vi "TraverseGObj.vi"(1 "Input":cluster{"Name":string, "Ctrl":refnum<vi>}[](array[cluster]), 2 "Prefix":string, 3 "GObj Reference":refnum<vi>) -> (0 "Output":cluster{"Name":string, "Ctrl":refnum<vi>}[](array[cluster]))   [LabVIEW 2014]
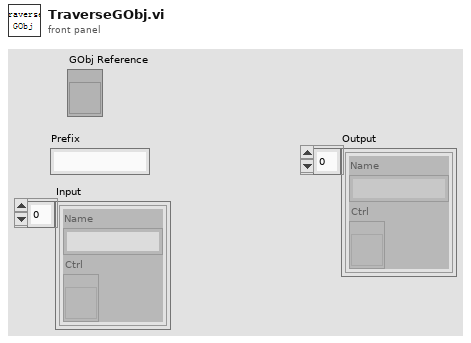
[diagram p1: front panel]
types:
  T1 = cluster{"Name":string, "GObj Reference":refnum<vi>}[]
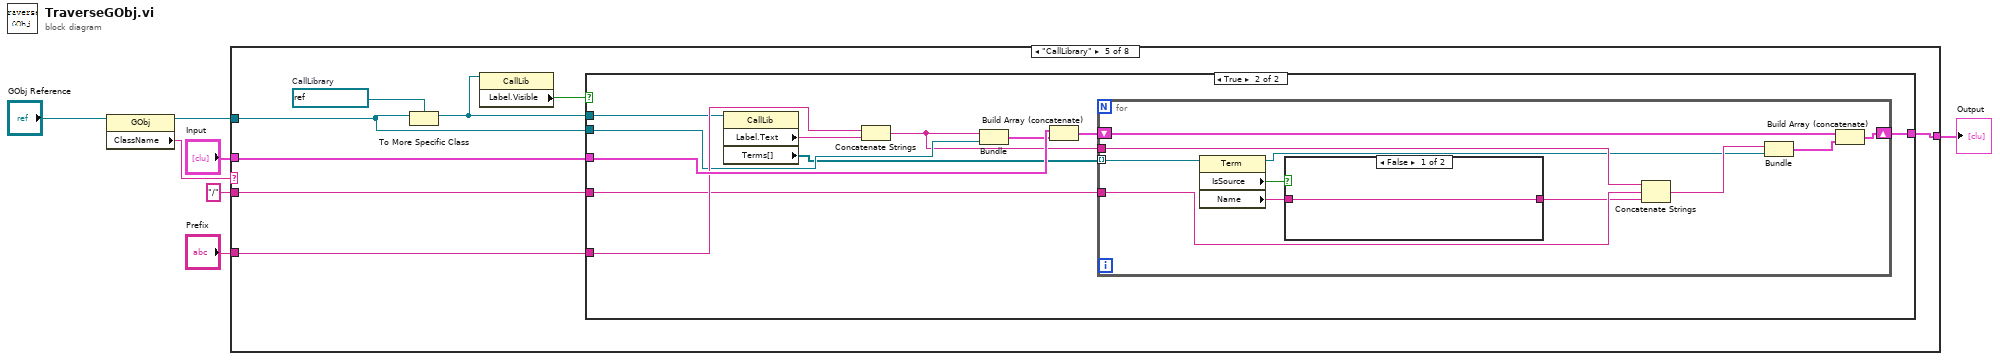
[diagram p0: block diagram]
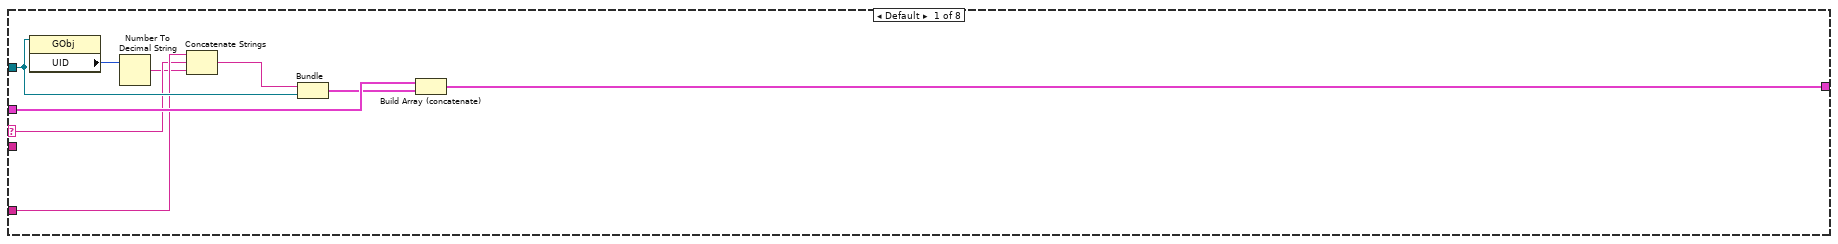
[diagram p2: hidden frame]
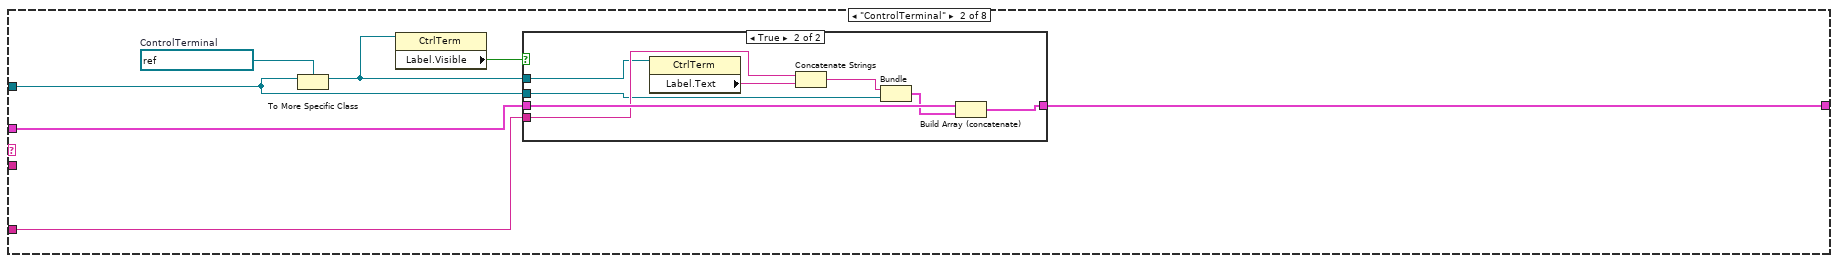
[diagram p3: hidden frame]
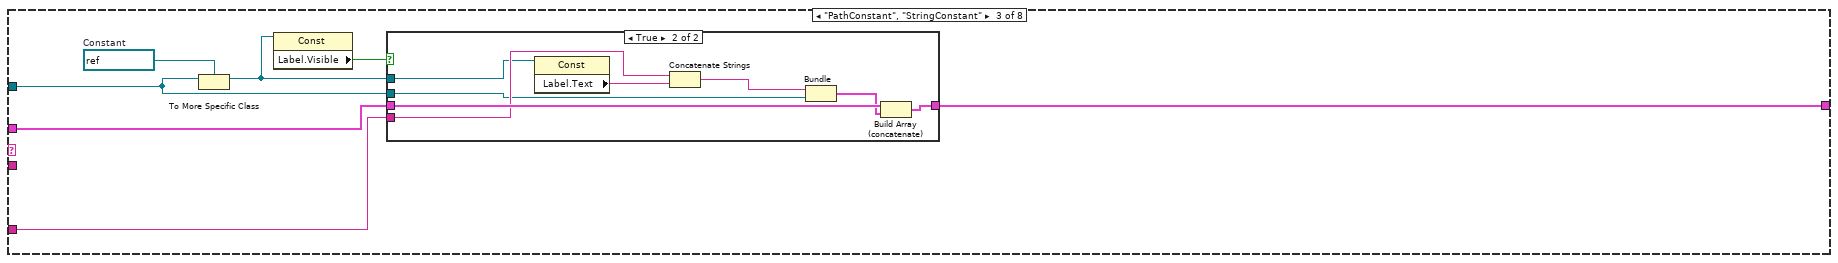
[diagram p5: hidden frame]
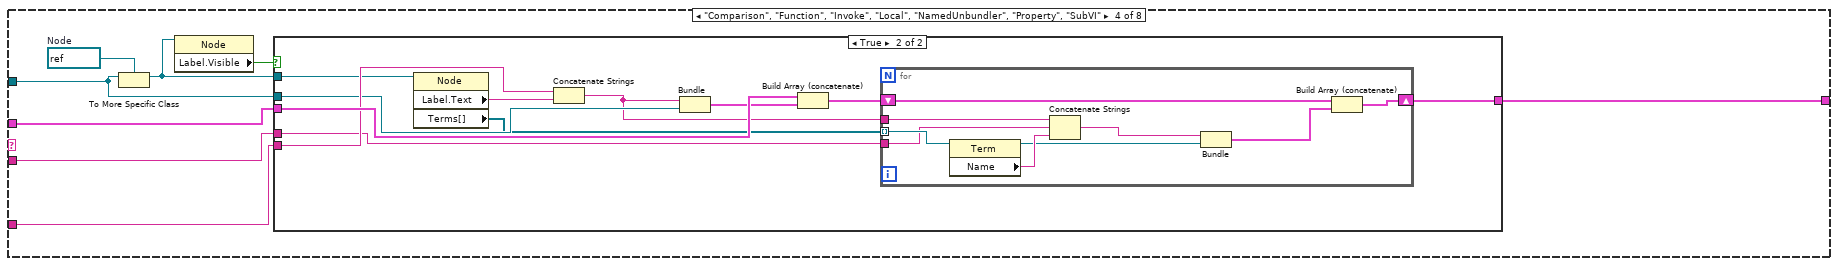
[diagram p7: hidden frame]
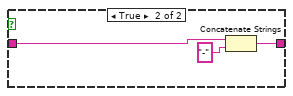
[diagram p10: hidden frame]
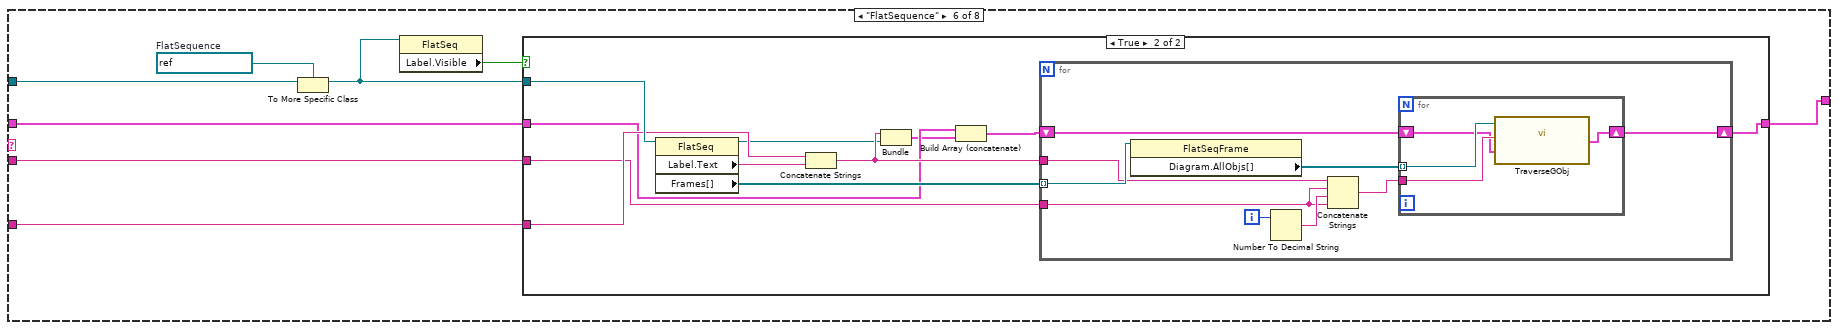
[diagram p11: hidden frame]
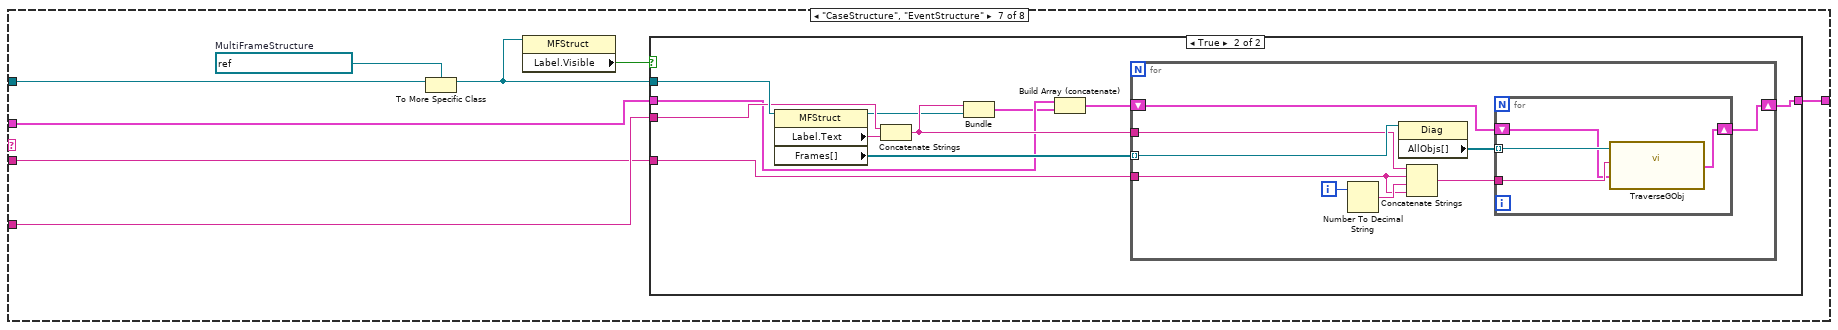
[diagram p13: hidden frame]
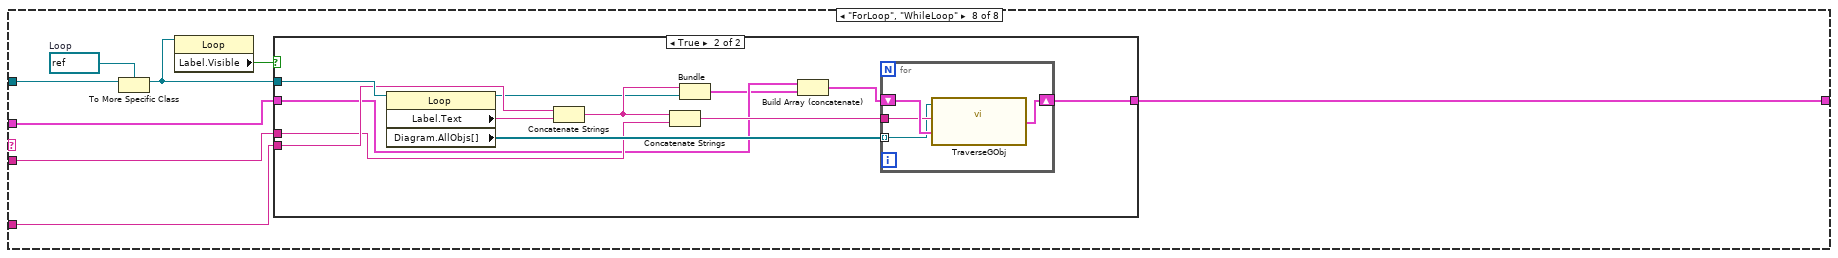
[diagram p15: hidden frame]
diagram:
  n1 = property on="Property Node" class="GObj"(reference="GObj Reference") -> (reference out=w6:refnum<vi>, "ClassName"=w7:string)  [unwired: 1 in, 1 out]
  n2 = case shown="\"CallLibrary\"" w7 {
    selector: w7 -> [w9 _ _ _ _ _ _ _]
    tunnel: w6 -> [w14 w19 w35 w52 w81 w120 w153 w186]
    tunnel: "Input" -> [w16 w23 w39 w56 w85 w118 w151 w185]
    tunnel: "Prefix" -> [w11 w21 w37 w54 w83 w117 w150 w184]
    tunnel: [w12 w22 w38 w55 w84 w116 w149 w183] -> w3
    tunnel: "/" ("string") -> [_ _ _ w49 w78 w115 w148 w181]
    frame Default {
      n3 = property class="GObj"(reference=w14) -> ("UID"=w13:i32)  [unwired: 1 in, 2 out]
      n4 = Number To Decimal String(number=w13) -> (decimal integer string=w8:string)  [unwired: 1 in]
      n5 = Concatenate Strings(w11, w9, w8) -> (w10:string)
      n6 = Bundle(w10, "GObj Reference"=w14) -> (w15:cluster{string, "GObj Reference":refnum<vi>})  [unwired: 1 in]
      n7 = Build Array (concatenate)(w16, w15) -> (w12:T1)
    }
    frame "ControlTerminal" {
      w20 = refnum<vi> refnum  # ControlTerminal
      n8 = To More Specific Class(target class=w20, reference=w19) -> (specific class reference=w18:refnum<vi>)  [unwired: 1 in, 1 out]
      n9 = property class="CtrlTerm"(reference=w18) -> ("Label.Visible"=w17:bool)  [unwired: 1 in, 2 out]
      n10 = case shown="True" w17 {
        tunnel: w23 -> [w24 w32]
        tunnel: [w24 w30] -> w22
        tunnel: w21 -> [_ w29]
        tunnel: w18 -> [_ w27]
        tunnel: w19 -> [_ w25]
        frame False {
        }
        frame True {
          n11 = property class="CtrlTerm"(reference=w27) -> ("Label.Text"=w26:string)  [unwired: 1 in, 2 out]
          n12 = Concatenate Strings(w29, w26) -> (w28:string)
          n13 = Bundle(w28, "GObj Reference"=w25) -> (w31:cluster{string, "GObj Reference":refnum<vi>})  [unwired: 1 in]
          n14 = Build Array (concatenate)(w32, w31) -> (w30:T1)
        }
      }
    }
    frame "PathConstant", "StringConstant" {
      w36 = refnum<vi> refnum  # Constant
      n15 = To More Specific Class(target class=w36, reference=w35) -> (specific class reference=w33:refnum<vi>)  [unwired: 1 in, 1 out]
      n16 = property class="Const"(reference=w33) -> ("Label.Visible"=w34:bool)  [unwired: 1 in, 2 out]
      n17 = case shown="True" w34 {
        tunnel: w39 -> [w40 w48]
        tunnel: [w40 w46] -> w38
        tunnel: w37 -> [_ w45]
        tunnel: w33 -> [_ w43]
        tunnel: w35 -> [_ w41]
        frame False {
        }
        frame True {
          n18 = property class="Const"(reference=w43) -> ("Label.Text"=w42:string)  [unwired: 1 in, 2 out]
          n19 = Concatenate Strings(w45, w42) -> (w44:string)
          n20 = Bundle(w44, "GObj Reference"=w41) -> (w47:cluster{string, "GObj Reference":refnum<vi>})  [unwired: 1 in]
          n21 = Build Array (concatenate)(w48, w47) -> (w46:T1)
        }
      }
    }
    frame "Comparison", "Function", "Invoke", "Local", "NamedUnbundler", "Property", "SubVI" {
      w53 = refnum<vi> refnum  # Node
      n22 = To More Specific Class(target class=w53, reference=w52) -> (specific class reference=w51:refnum<vi>)  [unwired: 1 in, 1 out]
      n23 = property class="Node"(reference=w51) -> ("Label.Visible"=w50:bool)  [unwired: 1 in, 2 out]
      n24 = case shown="True" w50 {
        tunnel: w56 -> [w57 w68]
        tunnel: [w57 w61] -> w55
        tunnel: w54 -> [_ w66]
        tunnel: w51 -> [_ w65]
        tunnel: w52 -> [_ w63]
        tunnel: w49 -> [_ w58]
        frame False {
        }
        frame True {
          n25 = property class="Node"(reference=w65) -> ("Label.Text"=w64:string, "Terms[]"=w60:refnum<vi>[])  [unwired: 1 in, 2 out]
          n26 = Concatenate Strings(w66, w64) -> (w59:string)
          n27 = Bundle(w59, "GObj Reference"=w63) -> (w67:cluster{string, "GObj Reference":refnum<vi>})  [unwired: 1 in]
          n28 = Build Array (concatenate)(w68, w67) -> (w62:T1)
          n29 = for {
            shift-right: [w69] -> w61
            shift-left: w62 -> [w71]
            tunnel: w60 -> [w77] mode=indexing
            tunnel: w59 -> [w76]
            tunnel: w58 -> [w75]
            n30 = property class="Term"(reference=w77) -> (reference out=w72:refnum<vi>, "Name"=w74:string)  [unwired: 1 in, 1 out]
            n31 = Concatenate Strings(w76, w75, w74) -> (w73:string)
            n32 = Bundle(w73, w72) -> (w70:cluster{string, refnum<vi>})  [unwired: 1 in]
            n33 = Build Array (concatenate)(w71, w70) -> (w69:T1)
          }
        }
      }
    }
    frame "CallLibrary" {
      w82 = refnum<vi> refnum  # CallLibrary
      n34 = To More Specific Class(target class=w82, reference=w81) -> (specific class reference=w80:refnum<vi>)  [unwired: 1 in, 1 out]
      n35 = property class="CallLib"(reference=w80) -> ("Label.Visible"=w79:bool)  [unwired: 1 in, 2 out]
      n36 = case shown="True" w79 {
        tunnel: w85 -> [w86 w97]
        tunnel: [w86 w90] -> w84
        tunnel: w83 -> [_ w95]
        tunnel: w80 -> [_ w94]
        tunnel: w81 -> [_ w92]
        tunnel: w78 -> [_ w87]
        frame False {
        }
        frame True {
          n37 = property class="CallLib"(reference=w94) -> ("Label.Text"=w93:string, "Terms[]"=w89:refnum<vi>[])  [unwired: 1 in, 2 out]
          n38 = Concatenate Strings(w95, w93) -> (w88:string)
          n39 = Bundle(w88, "GObj Reference"=w92) -> (w96:cluster{string, "GObj Reference":refnum<vi>})  [unwired: 1 in]
          n40 = Build Array (concatenate)(w97, w96) -> (w91:T1)
          n41 = for {
            shift-right: [w101] -> w90
            shift-left: w91 -> [w103]
            tunnel: w89 -> [w108] mode=indexing
            tunnel: w88 -> [w107]
            tunnel: w87 -> [w106]
            n42 = property class="Term"(reference=w108) -> (reference out=w104:refnum<vi>, "IsSource"=w100:bool, "Name"=w99:string)  [unwired: 1 in, 1 out]
            n43 = case shown="False" w100 {
              tunnel: w99 -> [w109 w112]
              tunnel: [w109 w110] -> w98
              frame False {
              }
              frame True {
                n44 = Concatenate Strings(w112, "-" ("string")) -> (w110:string)
              }
            }
            n45 = Concatenate Strings(w107, w106, w98) -> (w105:string)
            n46 = Bundle(w105, w104) -> (w102:cluster{string, refnum<vi>})  [unwired: 1 in]
            n47 = Build Array (concatenate)(w103, w102) -> (w101:T1)
          }
        }
      }
    }
    frame "FlatSequence" {
      w119 = refnum<vi> refnum  # FlatSequence
      n48 = To More Specific Class(target class=w119, reference=w120) -> (specific class reference=w114:refnum<vi>)  [unwired: 1 in, 1 out]
      n49 = property class="FlatSeq"(reference=w114) -> ("Label.Visible"=w113:bool)  [unwired: 1 in, 2 out]
      n50 = case shown="True" w113 {
        tunnel: w114 -> [_ w132]
        tunnel: w118 -> [w121 w124]
        tunnel: w117 -> [_ w131]
        tunnel: [w121 w128] -> w116
        tunnel: w115 -> [_ w127]
        frame False {
        }
        frame True {
          n51 = property class="FlatSeq"(reference=w132) -> (reference out=w125:refnum<vi>, "Label.Text"=w130:string, "Frames[]"=w129:refnum<vi>[])  [unwired: 1 in, 1 out]
          n52 = Concatenate Strings(w131, w130) -> (w126:string)
          n53 = Bundle(w126, w125) -> (w123:cluster{string, refnum<vi>})  [unwired: 1 in]
          n54 = Build Array (concatenate)(w124, w123) -> (w122:cluster{"Name":string, "Ctrl":refnum<vi>}[])
          n55 = for {
            tunnel: w129 -> [w141] mode=indexing
            tunnel: w126 -> [w140]
            shift-right: [w137] -> w128
            shift-left: w122 -> [w138]
            tunnel: w127 -> [w133]
            i -> [w135]
            n56 = property class="FlatSeqFrame"(reference=w141) -> ("Diagram.AllObjs[]"=w136:refnum<vi>[])  [unwired: 1 in, 2 out]
            n57 = Number To Decimal String(number=w135) -> (decimal integer string=w134:string)  [unwired: 1 in]
            n58 = Concatenate Strings(w140, w133, w134, w133) -> (w139:string)
            n59 = for {
              tunnel: w136 -> [w145] mode=indexing
              tunnel: w139 -> [w144]
              shift-right: [w142] -> w137
              shift-left: w138 -> [w143]
              n60 = call "TraverseGObj.vi"("Input"=w143, "Prefix"=w144, "GObj Reference"=w145) -> ("Output"=w142:cluster{"Name":string, "Ctrl":refnum<vi>}[])
            }
          }
        }
      }
    }
    frame "CaseStructure", "EventStructure" {
      w152 = refnum<vi> refnum  # MultiFrameStructure
      n61 = To More Specific Class(target class=w152, reference=w153) -> (specific class reference=w147:refnum<vi>)  [unwired: 1 in, 1 out]
      n62 = property class="MFStruct"(reference=w147) -> ("Label.Visible"=w146:bool)  [unwired: 1 in, 2 out]
      n63 = case shown="True" w146 {
        tunnel: w147 -> [_ w165]
        tunnel: w151 -> [w154 w157]
        tunnel: w150 -> [_ w164]
        tunnel: [w154 w161] -> w149
        tunnel: w148 -> [_ w160]
        frame False {
        }
        frame True {
          n64 = property class="MFStruct"(reference=w165) -> (reference out=w158:refnum<vi>, "Label.Text"=w163:string, "Frames[]"=w162:refnum<vi>[])  [unwired: 1 in, 1 out]
          n65 = Concatenate Strings(w164, w163) -> (w159:string)
          n66 = Bundle(w159, w158) -> (w156:cluster{string, refnum<vi>})  [unwired: 1 in]
          n67 = Build Array (concatenate)(w157, w156) -> (w155:cluster{"Name":string, "Ctrl":refnum<vi>}[])
          n68 = for {
            tunnel: w162 -> [w174] mode=indexing
            tunnel: w159 -> [w173]
            shift-right: [w170] -> w161
            shift-left: w155 -> [w171]
            tunnel: w160 -> [w166]
            i -> [w168]
            n69 = Number To Decimal String(number=w168) -> (decimal integer string=w167:string)  [unwired: 1 in]
            n70 = property class="Diag"(reference=w174) -> ("AllObjs[]"=w169:refnum<vi>[])  [unwired: 1 in, 2 out]
            n71 = Concatenate Strings(w173, w166, w167, w166) -> (w172:string)
            n72 = for {
              tunnel: w169 -> [w178] mode=indexing
              tunnel: w172 -> [w177]
              shift-right: [w175] -> w170
              shift-left: w171 -> [w176]
              n73 = call "TraverseGObj.vi"("Input"=w176, "Prefix"=w177, "GObj Reference"=w178) -> ("Output"=w175:cluster{"Name":string, "Ctrl":refnum<vi>}[])
            }
          }
        }
      }
    }
    frame "ForLoop", "WhileLoop" {
      w182 = refnum<vi> refnum  # Loop
      n74 = To More Specific Class(target class=w182, reference=w186) -> (specific class reference=w180:refnum<vi>)  [unwired: 1 in, 1 out]
      n75 = property class="Loop"(reference=w180) -> ("Label.Visible"=w179:bool)  [unwired: 1 in, 2 out]
      n76 = case shown="True" w179 {
        tunnel: w180 -> [_ w199]
        tunnel: w185 -> [w187 w190]
        tunnel: w184 -> [_ w198]
        tunnel: [w187 w196] -> w183
        tunnel: w181 -> [_ w194]
        frame False {
        }
        frame True {
          n77 = property class="Loop"(reference=w199) -> (reference out=w192:refnum<vi>, "Label.Text"=w197:string, "Diagram.AllObjs[]"=w195:refnum<vi>[])  [unwired: 1 in, 1 out]
          n78 = Concatenate Strings(w198, w197) -> (w193:string)
          n79 = Concatenate Strings(w193, w194) -> (w191:string)
          n80 = Bundle(w193, w192) -> (w189:cluster{string, refnum<vi>})  [unwired: 1 in]
          n81 = Build Array (concatenate)(w190, w189) -> (w188:cluster{"Name":string, "Ctrl":refnum<vi>}[])
          n82 = for {
            tunnel: w191 -> [w201]
            shift-right: [w202] -> w196
            shift-left: w188 -> [w203]
            tunnel: w195 -> [w200] mode=indexing
            n83 = call "TraverseGObj.vi"("Input"=w203, "Prefix"=w201, "GObj Reference"=w200) -> ("Output"=w202:cluster{"Name":string, "Ctrl":refnum<vi>}[])
          }
        }
      }
    }
  }
  "Output" <- w3
